vi "Puff_using_Arduino.vi"() -> (5 "Plug in titles":string[](array[string]), 7 "Plug in values":string[](array[string]))   [LabVIEW 2022 SP3]
uses:
  Globals/Meas_global.vi
panel:
  # "By selecting this vi to run you are telling Data Translation.vi to use the Puff with Arduino vi."
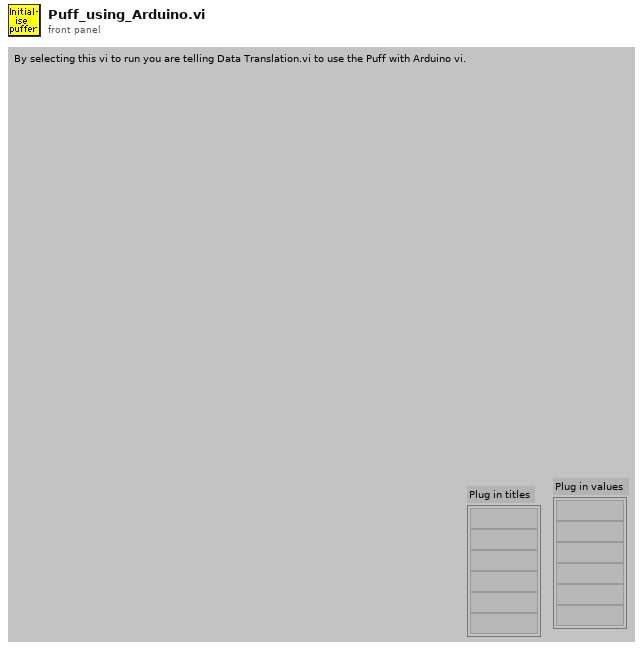
[diagram p1: front panel]
types:
  T1 = typedef "Post_Process.ctl" = enum16{"Take New Data", "Post Process Raw Data File"}
  T2 = typedef "Setup.ctl" = enum16{"Run Program", "Show Setup", "Save Current Setup", "Setup Front Panel"}
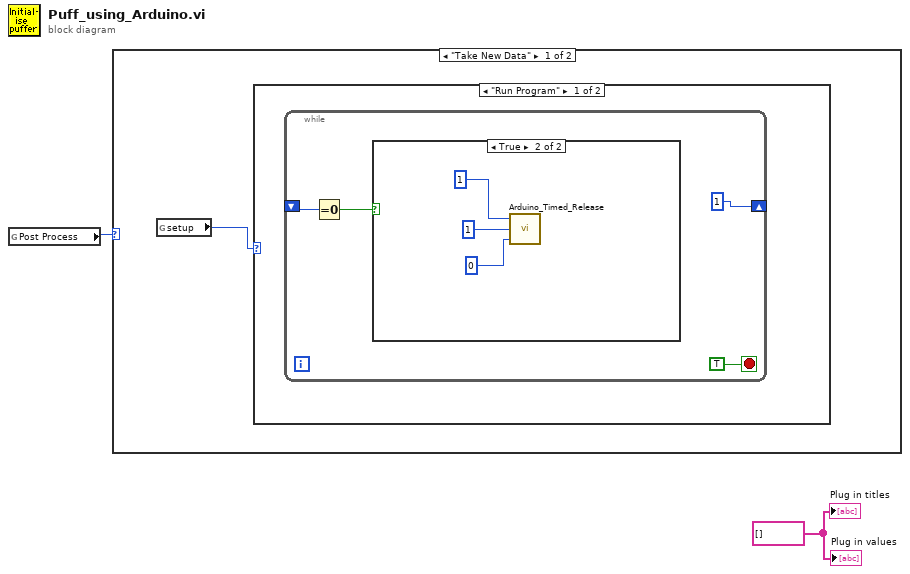
[diagram p0: block diagram]
diagram:
  w2 = string[] [] ("Plug in titles")
  n1 = global read "Meas_global.vi" "Post Process"() -> (w1:T1)
  n2 = case shown="\"Take New Data\"" w1 {
    frame "Take New Data" {
      n3 = global read "Meas_global.vi" "setup"() -> (w3:T2)
      n4 = case shown="\"Run Program\"" w3 {
        frame "Run Program" {
          n5 = while {
            shift-right: [1] -> _
            shift-left: _ -> [w6]
            stop <- TRUE stop-if-true
            n6 = Equal To 0?(x=w6) -> (x = 0?=w5:bool)
            n7 = case shown="True" w5 {
              frame False {
              }
              frame True {
                n8 = call "Arduino_Timed_Release.vi"("Time to hold source ON (microseconds)"=u32 0 ("Time to hold source OFF (microseconds)"), "Time to hold source OFF (microseconds)"=u32 1, "Number of cycles"=u16 1) -> ()  [unwired: 2 out]
              }
            }
          }
        }
        frame Default {
        }
      }
    }
    frame "Post Process Raw Data File" {
    }
  }
  "Plug in values" <- w2
  "Plug in titles" <- w2
